vi "TestBed.vi"() -> ()   [LabVIEW 2015]
uses:
  <vilib>/addons/h5labview/H5F_mode.ctl
  FPGA3/Limits_In.ctl
  User Interface/Controls/Role ID.ctl
  <userlib>/_OpenG.lib/file/file.llb/Build Path - Traditional__ogtk.vi
  <userlib>/_OpenG.lib/array/array.llb/Conditional Auto-Indexing Tunnel (String)__ogtk.vi
  <vilib>/addons/h5labview/polymorph/H5A_read_var.vi
  <vilib>/addons/database/_DB Variant To Data/Database Variant To Data.xnode
  <vilib>/addons/h5labview/H5File.lvlib
  <vilib>/addons/h5labview/H5GroupObject.lvlib
  <vilib>/addons/h5labview/H5Attrib.lvlib
panel:
  out "Speed Bracket":i32
  out "V-M-C Error":sgl[](array[numeric])
  in  "Dust ID":i32
  out "Waveform Graph":sgl[][](graph)
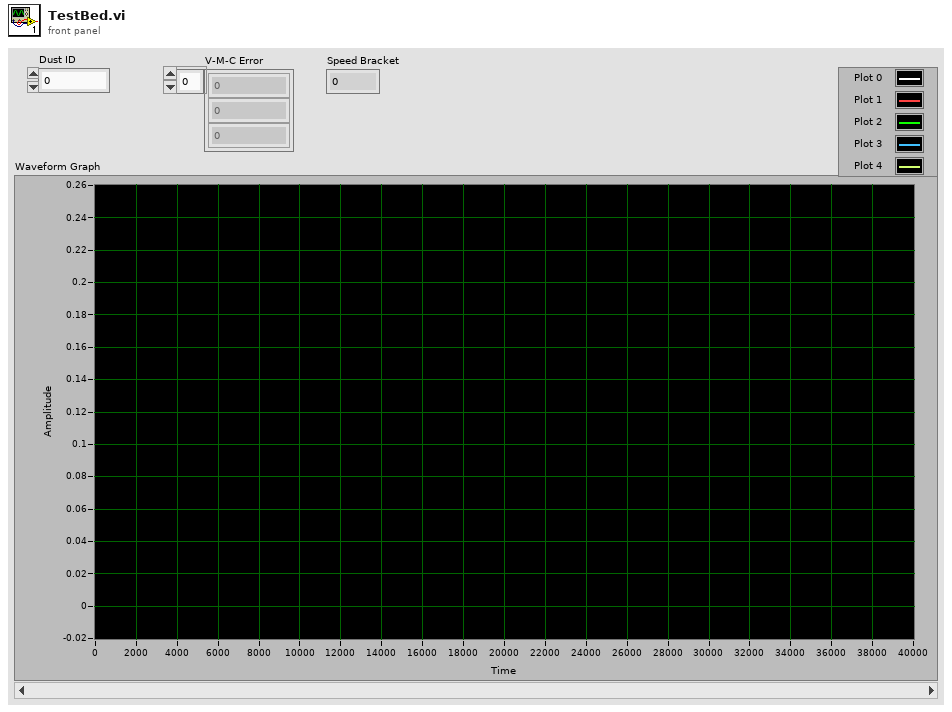
[diagram p1: front panel]
types:
  T1 = typedef "Role ID.ctl" = enum16{"First_Detector", "Second_Detector", "Third_Detector", "LeCroy_CH1", "LeCroy_CH2", "LeCroy_CH3", "LeCroy_CH4", "PSU", "DCS 1", "DCS 2"}
  T2 = typedef "Limits_In.ctl" = cluster{"High Charge Limit":fxp<+,32,-41>, "Low Charge Limit":fxp<+,32,-41>, "High Velocity Limit":fxp<+,18,18>, "Low Velocity Limit":fxp<+,18,18>, "High Mass Limit":fxp<+/-,33,-36>, "Low Mass Limit":fxp<+/-,33,-36>, "High Voltage":fxp<+,32,22>}
  T3 = typedef "H5File.lvlib/H5F_mode.ctl" = enum16{"read-only", "read-write", "overwrite", "create new", "open or create"}
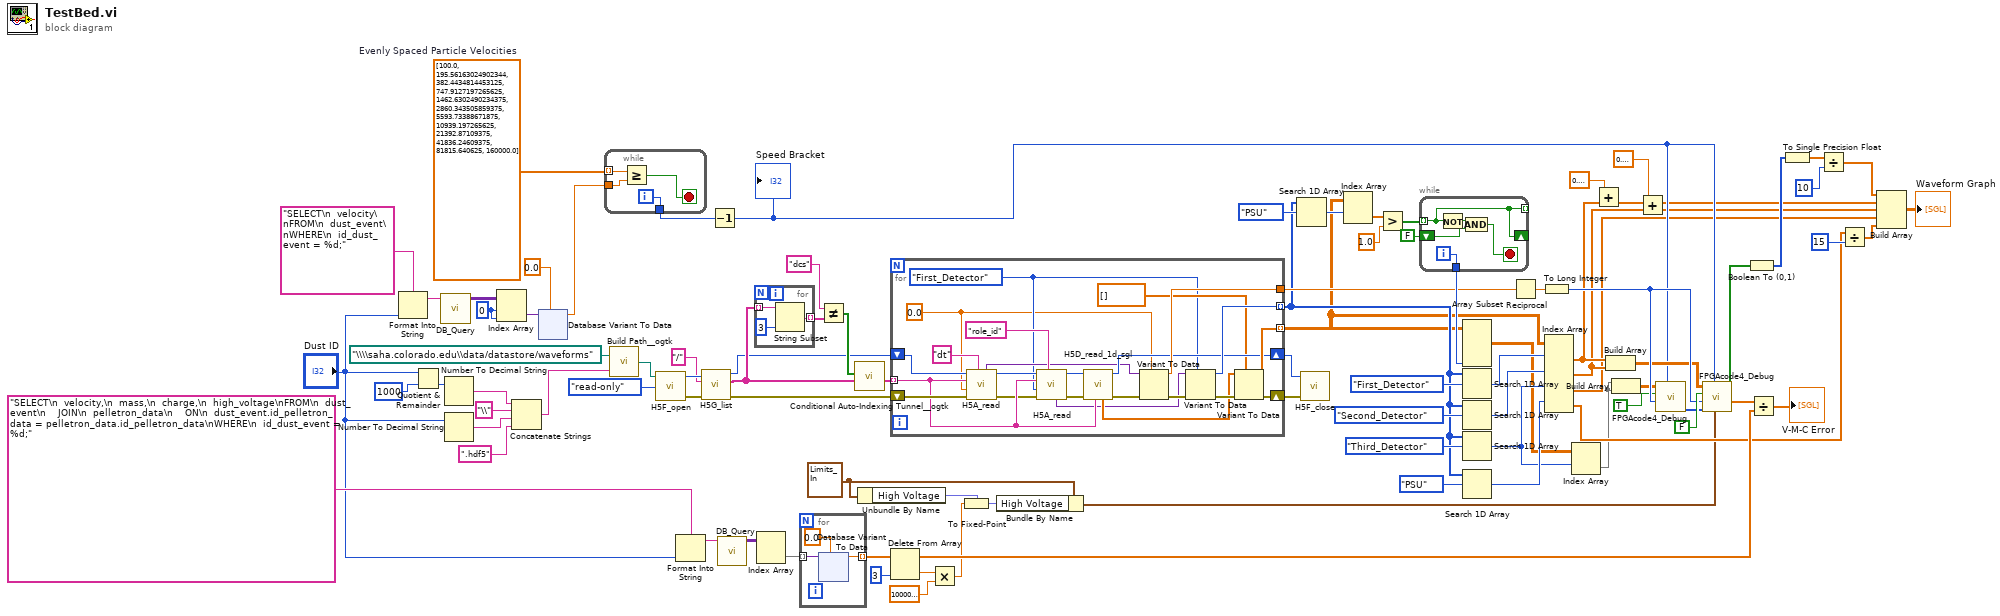
[diagram p0: block diagram]
diagram:
  w59 = T2 {"High Charge Limit"=4.54747350780585e-13, "Low Charge Limit"=0.0, "High Velocity Limit"=262143.0, "Low Velocity Limit"=0.0, "High Mass Limit"=7.27595761248936e-12, "Low Mass Limit"=0.0, "High Voltage"=2200000.0} ("Limits")
  w65 = sgl[] [100.0, 195.56163, 382.44348, 747.9127, 1462.6302, 2860.3435, 5593.734, 10939.197, 21392.871, 41836.246, 81815.64, 160000.0]  # Evenly Spaced Particle Velocities
  w69 = 0 ("index (row)")
  n1 = Format Into String(format string="SELECT\n  velocity\nFROM\n  dust_event\nWHERE\n  id_dust_event = %d;" ("Parameterized Query"), "Dust ID") -> (resulting string=w72:string)  [unwired: 2 in, 1 out]
  n2 = Quotient & Remainder(x="Dust ID", y=1000) -> (floor(x/y)=w75:i32)  [unwired: 1 out]
  n3 = call "DB_Query.vi"("Parameterized Query"=w72) -> ("Results"=w70:variant[][])  [unwired: 8 in, 2 out]
  n4 = Number To Decimal String(number=w75) -> (decimal integer string=w77:string)  [unwired: 1 in]
  n5 = Number To Decimal String(number="Dust ID") -> (decimal integer string=w79:string)  [unwired: 1 in]
  n6 = Index Array(array=w70, index (row)=w69, index (col)=w69) -> (element=w68:variant)
  n7 = Concatenate Strings(w77, "\\" ("string"), w79, ".hdf5" ("string")) -> (w73:string)
  n8 = xnode "Database Variant To Data"("database variant"=w68, "type"=sgl 0.0) -> ("data"=w66:sgl)  [unwired: 1 in, 1 out]
  n9 = while {
    tunnel: w66 -> [w95]
    tunnel: w65 -> [w96] mode=indexing
    tunnel: [w94] -> w64
    i -> [w94]
    stop <- w93 stop-if-true
    n10 = Greater Or Equal?(x=w96, y=w95) -> (x >= y?=w93:bool)
  }
  n11 = call-poly <userlib>:"Build Path__ogtk.vi"("name or relative path"=w73, "base path"=path "\\\\saha.colorado.edu\\data/datastore/waveforms") -> ("appended path"=w91:path)
  n12 = call <vilib>:"H5F_open.vi"("mode"=H5F_mode."read-only", "path"=w91) -> ("error out"=w89:errorcluster, "ref"=w90:i32)  [unwired: 2 in]
  n13 = Format Into String(format string="SELECT\n  velocity,\n  mass,\n  charge,\n  high_voltage\nFROM\n  dust_event\n    JOIN\n  pelletron_data\n    ON\n  dust_event.id_pelletron_data = pelletron_data.id_pelletron_data\nWHERE\n  id_dust_event = %d;" ("Parameterized Query"), "Dust ID") -> (resulting string=w63:string)  [unwired: 2 in, 1 out]
  n14 = call <vilib>:"H5G_list.vi"("error in (no error)"=w89, "group"="/", "ref"=w90) -> ("error out"=w25:errorcluster, "names"=w24:string[], "ref out"=w23:i32)  [unwired: 1 in, 1 out]
  n15 = Decrement(x=w64) -> (x-1=w22:i32)
  "Speed Bracket" <- w22
  n16 = call "DB_Query.vi"("Parameterized Query"=w63) -> ("Results"=w61:variant[][])  [unwired: 8 in, 2 out]
  n17 = for {
    tunnel: w24 -> [w98] mode=indexing
    tunnel: [w97] -> w44 mode=indexing
    n18 = String Subset(string=w98, length (rest)=3 ("length (rest)")) -> (substring=w97:string)  [unwired: 1 in]
  }
  n19 = Index Array(array=w61) -> (element=w60:variant[])  [unwired: 2 in]
  n20 = for {
    tunnel: w60 -> [w101] mode=indexing
    tunnel: [w100] -> w58 mode=indexing
    n21 = xnode "Database Variant To Data"("database variant"=w101, "type"=sgl 0.0) -> ("data"=w100:sgl)  [unwired: 1 in, 1 out]
  }
  n22 = Not Equal?(x="dcs" ("y"), y=w44) -> (x != y?=w43:bool[])
  n23 = call-poly <userlib>:"Conditional Auto-Indexing Tunnel__ogtk.vi"("Array in"=w24, "Elements to keep"=w43) -> ("Filtered Array out"=w42:string[])  [unwired: 5 in]
  n24 = Unbundle By Name(w59) -> ("High Voltage"=w54:fxp<+,32,22>)
  n25 = for {
    shift-right: [w146] -> w40
    shift-left: w25 -> [w150]
    shift-right: [w144] -> w41
    shift-left: w23 -> [w151]
    tunnel: [w153] -> w15 mode=indexing
    tunnel: [w154] -> w1 mode=indexing
    tunnel: [w149] -> w32
    tunnel: w42 -> [w143] mode=indexing
    w136 = 0.0
    w137 = Role_ID."First_Detector" ("Role ID")
    n26 = call-poly <vilib>:"H5A_read.vi"("attrib_name"="dt", "error in (no error)"=w150, "default"=w136, "obj_name"=w143, "ref"=w151) -> ("error out"=w139:errorcluster, "ref out"=w145:i32, "value"=w141:variant)  [unwired: 2 in]
    n27 = call-poly <vilib>:"H5A_read.vi"("attrib_name"="role_id", "error in (no error)"=w139, "default"=w137, "obj_name"=w143, "ref"=w145) -> ("error out"=w138:errorcluster, "ref out"=w155:i32, "value"=w140:variant)  [unwired: 2 in]
    n28 = call "H5D_read_1d_sgl.vi"("name"=w143, "error in (no error)"=w138, "ref"=w155) -> ("error out"=w135:errorcluster, "ref out"=w144:i32, "data"=w152:sgl[])  [unwired: 4 in]
    n29 = Variant To Data(error in=w135, type=w136, Variant=w141) -> (data=w149:dbl, error out=w147:errorcluster)
    n30 = Variant To Data(error in=w147, type=w137, Variant=w140) -> (data=w153:T1, error out=w156:errorcluster)
    n31 = Variant To Data(error in=w156, type=sgl[] [] ("Data"), Variant=w152) -> (data=w154:sgl[], error out=w146:errorcluster)
  }
  n32 = Delete From Array(array=w58, index=3) -> (deleted portion=w56:sgl, array with subset deleted=w53:sgl[])  [unwired: 1 in]
  n33 = Multiply(x=w56, y=sgl 1000000.0) -> (x*y=w51:sgl)
  n34 = To Fixed-Point(fixed-point type=w54, number=w51) -> (fixed-point=w55:fxp<+,32,22>)
  n35 = Bundle By Name(cluster=w59, "High Voltage"=w55) -> (w12:T2)
  n36 = Search 1D Array(1D array=w15, element=Role_ID."PSU") -> (index of element=w36:i32)  [unwired: 1 in]
  n37 = call <vilib>:"H5F_close.vi"("error in (no error)"=w40, "ref"=w41) -> ()  [unwired: 3 in, 1 out]
  n38 = Index Array(array=w1, index (row)=w36) -> (element=w38:sgl[])  [unwired: 1 in]
  n39 = Greater?(x=w38, y=sgl 1.0) -> (0:w6:bool[])
  n40 = while {
    tunnel: w6 -> [w158] mode=indexing
    shift-right: [w158] -> _
    shift-left: FALSE -> [w161]
    tunnel: [w160] -> w46
    tunnel: [w158] -> _ mode=indexing
    i -> [w160]
    stop <- w159 stop-if-true
    n41 = Not(x=w158) -> (.not. x?=w162:bool)
    n42 = And(x=w162, y=w161) -> (x .and. y?=w159:bool)
  }
  n43 = Array Subset(array=w1, length (col)=w46) -> (w2:sgl[][])  [unwired: 3 in]
  n44 = Search 1D Array(1D array=w15, element=Role_ID."First_Detector") -> (index of element=w47:i32)  [unwired: 1 in]
  n45 = Search 1D Array(1D array=w15, element=Role_ID."Second_Detector") -> (index of element=w48:i32)  [unwired: 1 in]
  n46 = Search 1D Array(1D array=w15, element=Role_ID."Third_Detector") -> (index of element=w4:i32)  [unwired: 1 in]
  n47 = Search 1D Array(1D array=w15, element=Role_ID."PSU") -> (index of element=w14:i32)  [unwired: 1 in]
  n48 = Reciprocal(x=w32) -> (1/x=w33:dbl)
  n49 = To Long Integer(number=w33) -> (32bit integer=w34:i32)
  n50 = Index Array(array=w1, index (row) #1=w47, index (row) #2=w48, index (row) #3=w4, index (row) #4=w14) -> (element #1=w19:sgl[], element #2=w18:sgl[], element #3=w17:sgl[], element #4=w13:sgl[])  [unwired: 4 in]
  n51 = Index Array(array=w2, index (row)=w4) -> (element=w3:sgl[])  [unwired: 1 in]
  n52 = Add(x=sgl 0.2, y=w19) -> (x+y=w11:sgl[])
  n53 = Build Array(w19, w18) -> (w29:sgl[][])
  n54 = Build Array(w3, w3) -> (w31:sgl[][])
  n55 = Add(x=sgl 0.1, y=w18) -> (x+y=w9:sgl[])
  n56 = call "FPGAcode4_Debug.vi"("Speed Bracket"=w22, "Clock Speed (Hz)"=w34, "Calibrate"=TRUE, "Detector Waveform In"=w31) -> ("Thresholds out"=w37:i32[])  [unwired: 4 in, 3 out]
  n57 = call "FPGAcode4_Debug.vi"("Limits"=w12, "Speed Bracket"=w22, "Thresholds in"=w37, "Clock Speed (Hz)"=w34, "Calibrate"=FALSE, "Detector Waveform In"=w29) -> ("V-M-C Estimate"=w21:sgl[], "PSU Response"=w20:bool[])  [unwired: 2 in, 2 out]
  n58 = Boolean To (0,1)(Boolean=w20) -> (0, 1=w87:i16[])
  n59 = Divide(x=w21, y=w53) -> (x/y=→"V-M-C Error":sgl[])
  n60 = To Single Precision Float(number=w87) -> (single precision float=w85:sgl[])
  n61 = Divide(x=w85, y=10) -> (x/y=w81:sgl[])
  n62 = Divide(x=w13, y=15) -> (x/y=w84:sgl[])
  n63 = Build Array(w81, w11, w9, w17, w84) -> (→"Waveform Graph":sgl[][])
